vi "Read Control Input Pot.vi"() -> ()   [LabVIEW 2014]
uses:
  <vilib>/rvi/Emulation/niFpgaGetClockAttributes.vi
  <vilib>/rvi/Emulation/niFpgaSctlEmulationGetInTimedLoop.vi
  <vilib>/rvi/Emulation/niFpgaEmulationReportErrorSimple.vi
  <vilib>/rvi/eio/common/nirviEmuTemplateMethod_errors.vi
  <vilib>/rvi/Emulation/niFpgaCriticalErrorInLSC.vi
  <vilib>/eio/EIONode/EIONode.xnode
panel:
  out "Angular Position":fxp<+/-,33,11>
  in  "stop":bool
  out "Boolean":bool
  out "Raw Setpoint Pot":fxp<+/-,16,5>
  in  "Count(mSec)":u32
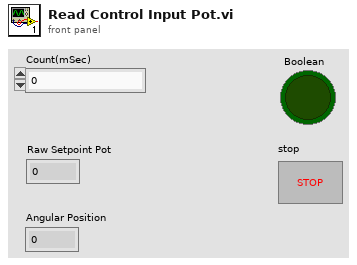
[diagram p1: front panel]
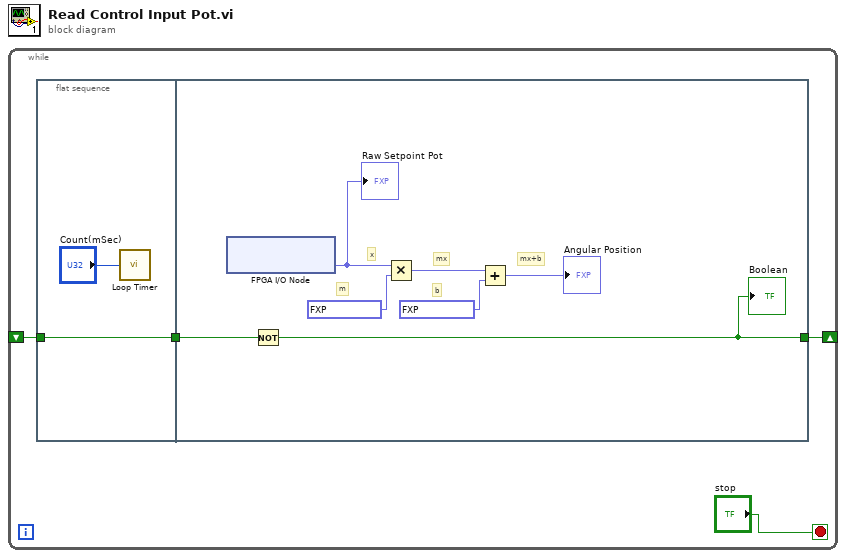
[diagram p0: block diagram]
diagram:
  n1 = while {
    shift-right: [w2] -> _
    shift-left: _ -> [w3]
    stop <- "stop" stop-if-true
    n2 = flat-sequence {
      tunnel: w3 -> [w5]
      tunnel: [w5] -> w4
      tunnel: w4 -> [w13]
      tunnel: [w12] -> w2
      frame #0 {
        n3 = call "Loop Timer"("Count(mSec)"="Count(mSec)") -> ()  [unwired: 1 out]
      }
      frame #1 {
        # "mx+b"
        # "x"
        # "mx"
        # "b"
        # "m"
        n4 = xnode "FPGA I/O Node"() -> ("Setpoint Pot"=w11:fxp<+/-,16,5>)  [unwired: 1 in, 1 out]
        "Raw Setpoint Pot" <- w11
        n5 = Not(x=w13) -> (.not. x?=w12:bool)
        "Boolean" <- w12
        n6 = Multiply(x=w11, y=fxp<+/-,17,6> -25.12890625) -> (x*y=w10:fxp<+/-,11,9>)
        n7 = Add(x=w10, y=fxp<+,17,9> 257.83984375) -> (x+y=→"Angular Position":fxp<+,11,9>)
      }
    }
  }
